vi "Processing Message Loop.vi"(8 "error in (no error)":errorcluster, 10 "Queue A - Processing":refnum<queue>, 11 "Message Queues":T1) -> (0 "error out":errorcluster)   [LabVIEW 2026, in "Processing_Engine.lvlib"]
doc: "The message loop subVI to handle messages pertaining to logging data."
uses:
  Processing_Engine.lvlib
  support/Architecture/Message Queue/All Message Queues.ctl
  support/Architecture/Message Queue/Message Cluster.ctl
  Processing Settings.ctl
  controls/Messaging Payloads/Sensor CoreData.ctl
  controls/Messaging Payloads/Sensor CoreData Cluster.ctl
  controls/UI/Units Enum.ctl
  controls/UI/Signal Enum.ctl
  Test Parameters.ctl
  Test Parameters Cluster.ctl
  controls/UI/Measurement Role.ctl
  controls/UI/Test Sequence Context.ctl
  controls/UI/Test Sequence Context Cluster.ctl
  controls/UI/Direction.ctl
  Processing State.ctl
  support/Architecture/Message Queue/Enqueue Message (Single).vi
  <vilib>/Utility/error.llb/Error Cluster From Error Code.vi
  <vilib>/ErrorRing/Error Ring.xnode
  support/Architecture/Message Queue/Message Queue.lvlib
  Settings/Settings.lvlib
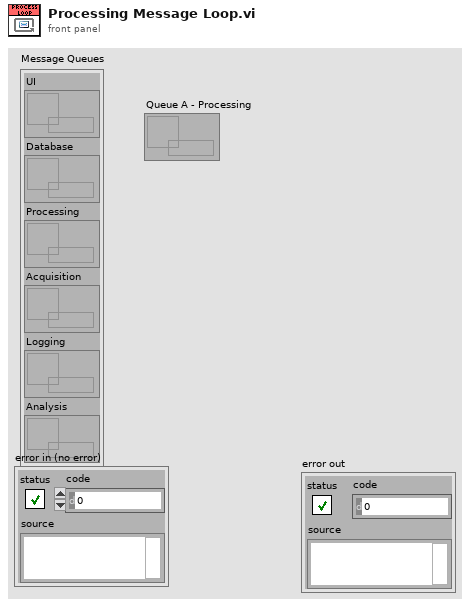
[diagram p1: front panel]
types:
  T1 = typedef "Message Queue.lvlib/All Message Queues.ctl" = cluster{"UI":refnum<queue>, "Database":refnum<queue>, "Processing":refnum<queue>, "Acquisition":refnum<queue>, "Logging":refnum<queue>, "Analysis":refnum<queue>}
  T2 = typedef "Processing_Engine.lvlib/Processing State.ctl" = enum16{"Idle", "Processing"}
  T3 = typedef "Processing_Engine.lvlib/Processing Settings.ctl" = cluster{"Sensor CoreData":T4, "Test Parameters":T8, "Measurement Roles":T10[], "Test Sequence Context":T11}
  T4 = typedef "Sensor CoreData.ctl" = T5[]
  T5 = typedef "Settings.lvlib/Sensor CoreData Cluster.ctl" = cluster{"SerialNumber":string, "ModelNumber":string, "Min":dbl, "Max":dbl, "Units":T6, "Output Signal":T7, "SensorID":i32}
  T6 = typedef "Units Enum.ctl" = enum16{"PSI", "Deg C", "kPa", "GPM"}
  T7 = typedef "Signal Enum.ctl" = enum16{"4-20mA", "0-10V", "Thermocouple Type K"}
  T8 = typedef "Processing_Engine.lvlib/Test Parameters.ctl" = T9[]
  T9 = typedef "Settings.lvlib/Test Parameters Cluster.ctl" = cluster{"Steady-State Duration (s)":i32, "Allowed Tolerance (%) FS":dbl, "Max Settling Timeout (s)":i32}
  T10 = typedef "Settings.lvlib/Measurement Role.ctl" = enum16{"Controller", "Reference", "UUT", "Disable", "All"}
  T11 = typedef "Settings.lvlib/Test Sequence Context.ctl" = T12[]
  T12 = typedef "Settings.lvlib/Test Sequence Context Cluster.ctl" = cluster{"Direction":T13, "Cycle Number":i32}
  T13 = typedef "Settings.lvlib/Direction.ctl" = enum16{"Acsending", "Descending"}
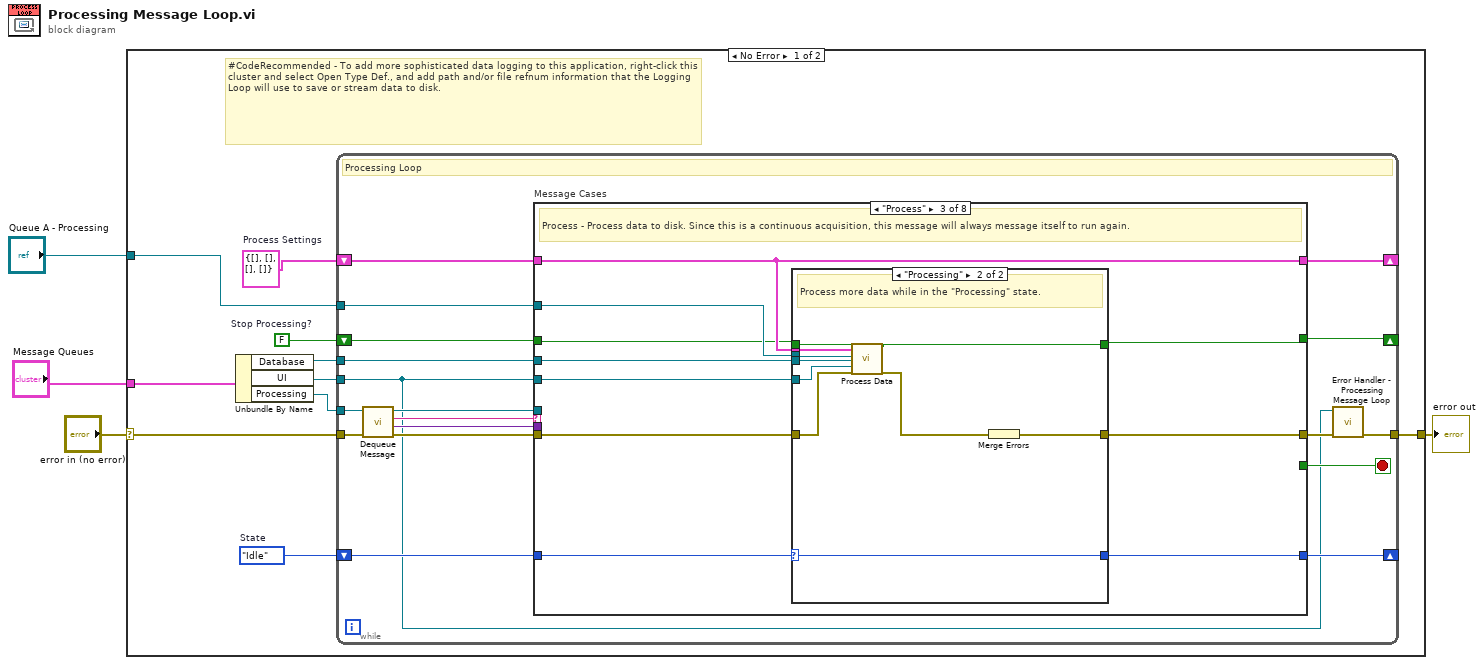
[diagram p0: block diagram]
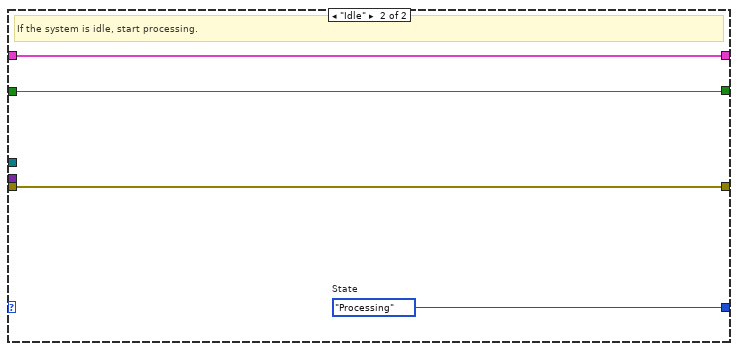
[diagram p4: hidden frame]
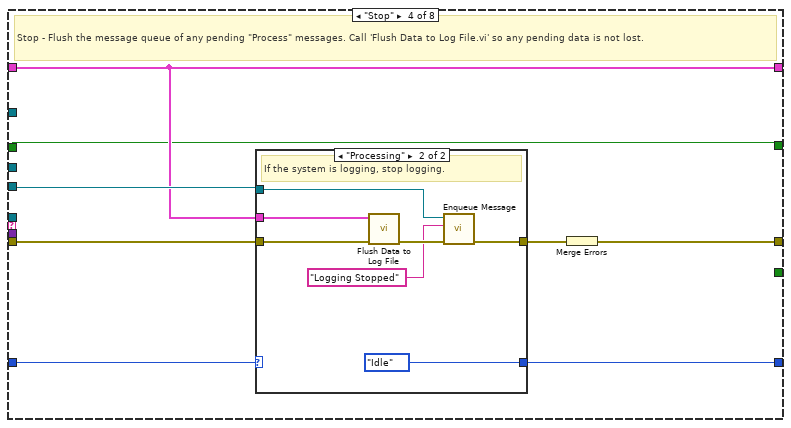
[diagram p6: hidden frame]
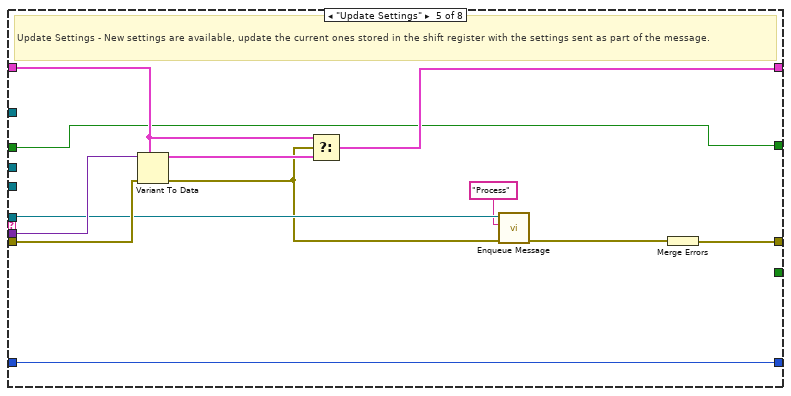
[diagram p8: hidden frame]
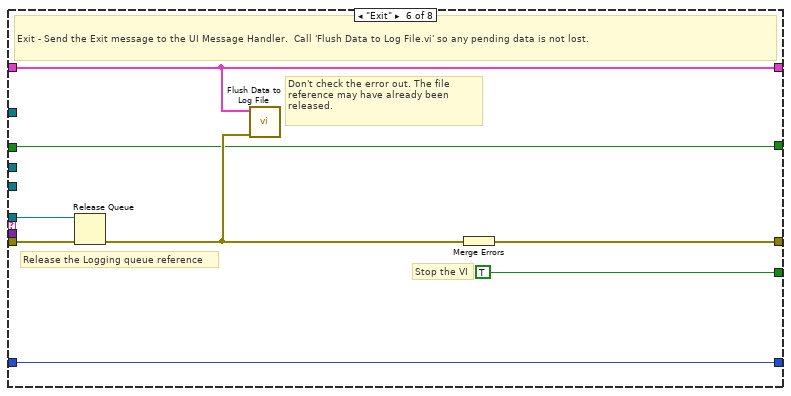
[diagram p9: hidden frame]
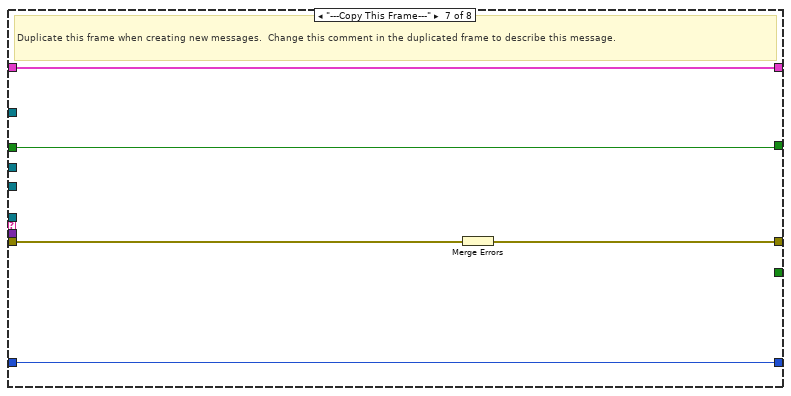
[diagram p10: hidden frame]
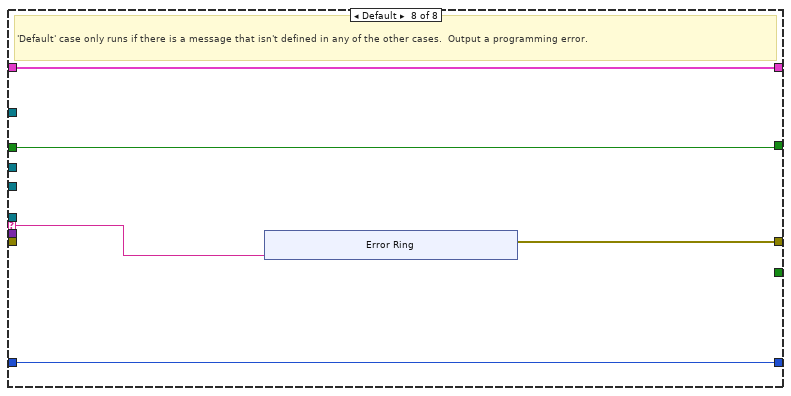
[diagram p11: hidden frame]
diagram:
  n1 = case shown="No Error" "error in (no error)" {
    selector: "error in (no error)" -> [w10 w132]
    tunnel: "Message Queues" -> [w14 _]
    tunnel: [w12 w132] -> w3
    tunnel: "Queue A - Processing" -> [w7 _]
    frame No Error {
      w5 = FALSE  # Stop Processing?
      w8 = Processing_State."Idle"  # State
      w11 = T3 {"Sensor CoreData"=[], "Test Parameters"=[], "Measurement Roles"=[], "Test Sequence Context"=[]}  # Process Settings
      # "#CodeRecommended - To add more sophisticated data logging to this application, right-click this cluster and select Open Type Def., and add path and/or file refnum information that the Logging Loop will use to save or stream data to disk."
      n2 = Unbundle By Name(w14) -> ("Database"=w6:refnum<queue>, "UI"=w9:refnum<queue>, "Processing"=w13:refnum<queue>)
      n3 = while {
        tunnel: w13 -> [w24]
        shift-right: [w31] -> _
        shift-left: w11 -> [w32]
        tunnel: w9 -> [w19]
        shift-right: [w22] -> _
        shift-left: w8 -> [w23]
        tunnel: w10 -> [w29]
        tunnel: [w21] -> w12
        tunnel: w7 -> [w18]
        tunnel: w6 -> [w17]
        shift-right: [w16] -> _
        shift-left: w5 -> [w15]
        stop <- w30 stop-if-true
        # "Processing Loop"
        n4 = call "Dequeue Message.vi"("error in (no error)"=w29, "Message Queue"=w24) -> ("error out"=w28:errorcluster, "Message Data"=w26:variant, "Message"=w27:string, "dup Message Queue"=w25:refnum<queue>)  [unwired: 6 in]
        n5 = case "Message Cases" shown="\"Process\"" w27 {
          selector: w27 -> [_ _ _ _ _ _ _ w121]
          tunnel: w25 -> [_ w45 _ _ w98 w111 _ _]
          tunnel: w28 -> [w35 w44 w63 w83 w101 w112 w119 _]
          tunnel: [w35 w46 w64 w85 w106 w113 w117 w122] -> w20
          tunnel: w32 -> [w36 w43 w62 w79 w104 w109 w118 w124]
          tunnel: [w36 w42 w62 w79 w102 w109 w118 w124] -> w31
          tunnel: [_ _ _ _ _ TRUE _ _] -> w30
          tunnel: w26 -> [_ w39 _ _ w105 _ _ _]
          tunnel: w19 -> [_ _ w57 w80 _ _ _ _]
          tunnel: w23 -> [w34 w41 w61 w82 w100 w108 w116 w123]
          tunnel: [w34 w40 w60 w81 w100 w108 w116 w123] -> w22
          tunnel: w18 -> [_ _ w59 _ _ _ _ _]
          tunnel: w17 -> [_ _ w58 _ _ _ _ _]
          tunnel: [w33 w37 w56 w78 w99 w107 w115 w120] -> w16
          tunnel: w15 -> [w33 w38 w55 w78 w99 w107 w115 w120]
          frame "Initialize" {
            # "Initialize - gets called when first launched. Currently a no-op."
          }
          frame "Start" {
            # "Start - Send the \"Process\" message to start processing."
            n6 = case shown="\"Processing\"" w41 {
              selector: w41 -> [w49 _]
              tunnel: [w48 w51] -> w46
              tunnel: w45 -> [_ _]
              tunnel: w44 -> [w48 w51]
              tunnel: w43 -> [w50 w53]
              tunnel: [w50 w53] -> w42
              tunnel: [w49 w54] -> w40
              tunnel: w39 -> [_ _]
              tunnel: w38 -> [w47 w52]
              tunnel: [w47 w52] -> w37
              frame "Processing" {
                # "The system is already processing. Ignore the \"Start\" message."
              }
              frame "Idle" {
                w54 = Processing_State."Processing"  # State
                # "If the system is idle, start processing."
              }
            }
          }
          frame "Process" {
            # "Process - Process data to disk. Since this is a continuous acquisition, this message will always message itself to run again."
            n7 = case shown="\"Processing\"" w61 {
              selector: w61 -> [w67 w74]
              tunnel: [w66 w77] -> w64
              tunnel: w63 -> [w66 w68]
              tunnel: w62 -> [_ w75]
              tunnel: [w67 w74] -> w60
              tunnel: w59 -> [_ w73]
              tunnel: w58 -> [_ w72]
              tunnel: w57 -> [_ w71]
              tunnel: [w65 w70] -> w56
              tunnel: w55 -> [w65 w69]
              frame "Idle" {
                # "Ignore \"Log\" messages when the logging is idle."
              }
              frame "Processing" {
                # "Process more data while in the \"Processing\" state."
                n8 = call "Process Data.vi"("Execution Flag in"=w69, "Processing Configuration"=w75, "Queue A - Processing"=w73, "Database"=w72, "UI"=w71, "error in (no error)"=w68) -> ("Stop Processing?"=w70:bool, "error out"=w76:errorcluster)  [unwired: 12 in]
                n9 = Merge Errors(w76) -> (w77:errorcluster)
              }
            }
          }
          frame "Stop" {
            # "Stop - Flush the message queue of any pending \"Process\" messages. Call 'Flush Data to Log File.vi' so any pending data is not lost."
            n10 = case shown="\"Processing\"" w82 {
              selector: w82 -> [w86 _]
              tunnel: [w87 w90] -> w84
              tunnel: w79 -> [_ w93]
              tunnel: w83 -> [w87 w92]
              tunnel: [w86 Processing_State."Idle" ("State")] -> w81
              tunnel: w80 -> [_ w89]
              frame "Idle" {
                # "The system is already idle. Ignore the \"Stop\" message."
              }
              frame "Processing" {
                # "If the system is logging, stop logging."
                n11 = call "Flush Data to Log File.vi"("error in (no error)"=w92, "Logging Configuration"=w93) -> ("error out"=w94:errorcluster)  [unwired: 9 in]
                n12 = call-poly "Enqueue Message.vi"("error in (no error)"=w94, "Message"="Logging Stopped", "Message Queue"=w89) -> ("error out"=w90:errorcluster)  [unwired: 7 in, 1 out]
              }
            }
            n13 = Merge Errors(w84) -> (w85:errorcluster)
          }
          frame "Update Settings" {
            # "Update Settings - New settings are available, update the current ones stored in the shift register with the settings sent as part of the message."
            n14 = Variant To Data(error in=w101, type=w104, Variant=w105) -> (data=w103:T3, error out=w96:errorcluster)
            n15 = Select(t=w104, s=w96, f=w103) -> (s? t:f=w102:T3)
            n16 = call-poly "Enqueue Message.vi"("error in (no error)"=w96, "Message"="Process", "Message Queue"=w98) -> ("error out"=w95:errorcluster)  [unwired: 7 in, 1 out]
            n17 = Merge Errors(w95) -> (w106:errorcluster)
          }
          frame "Exit" {
            # "Don't check the error out. The file reference may have already been released."
            # "Release the Logging queue reference"
            # "Stop the VI"
            # "Exit - Send the Exit message to the UI Message Handler.  Call 'Flush Data to Log File.vi' so any pending data is not lost."
            n18 = Release Queue(queue=w111, error in (no error)=w112) -> (error out=w110:errorcluster)  [unwired: 1 in, 2 out]
            n19 = call "Flush Data to Log File.vi"("error in (no error)"=w110, "Logging Configuration"=w109) -> ()  [unwired: 9 in, 1 out]
            n20 = Merge Errors(w110) -> (w113:errorcluster)
          }
          frame "---Copy This Frame---" {
            # "Duplicate this frame when creating new messages.  Change this comment in the duplicated frame to describe this message."
            n21 = Merge Errors(w119) -> (w117:errorcluster)
          }
          frame Default {
            # "'Default' case only runs if there is a message that isn't defined in any of the other cases.  Output a programming error."
            n22 = xnode "Error Ring"("parameter 0"=w121) -> ("error out"=w122:errorcluster)
          }
        }
        n23 = call "Error Handler - Processing Message Loop.vi"("error in (no error)"=w20, "Message Queue"=w19) -> ("dup error in"=w21:errorcluster)  [unwired: 8 in, 1 out]
      }
    }
    frame Error {
    }
  }
  "error out" <- w3
